vi "image acquisition practice2fail.vi"() -> ()   [LabVIEW 2014]
uses:
  <vilib>/vision/Image Controls.llb/IMAQ Image.ctl
panel:
  out "Circular Particles":T1
  out "Image Acquired":T1(plugin-control)
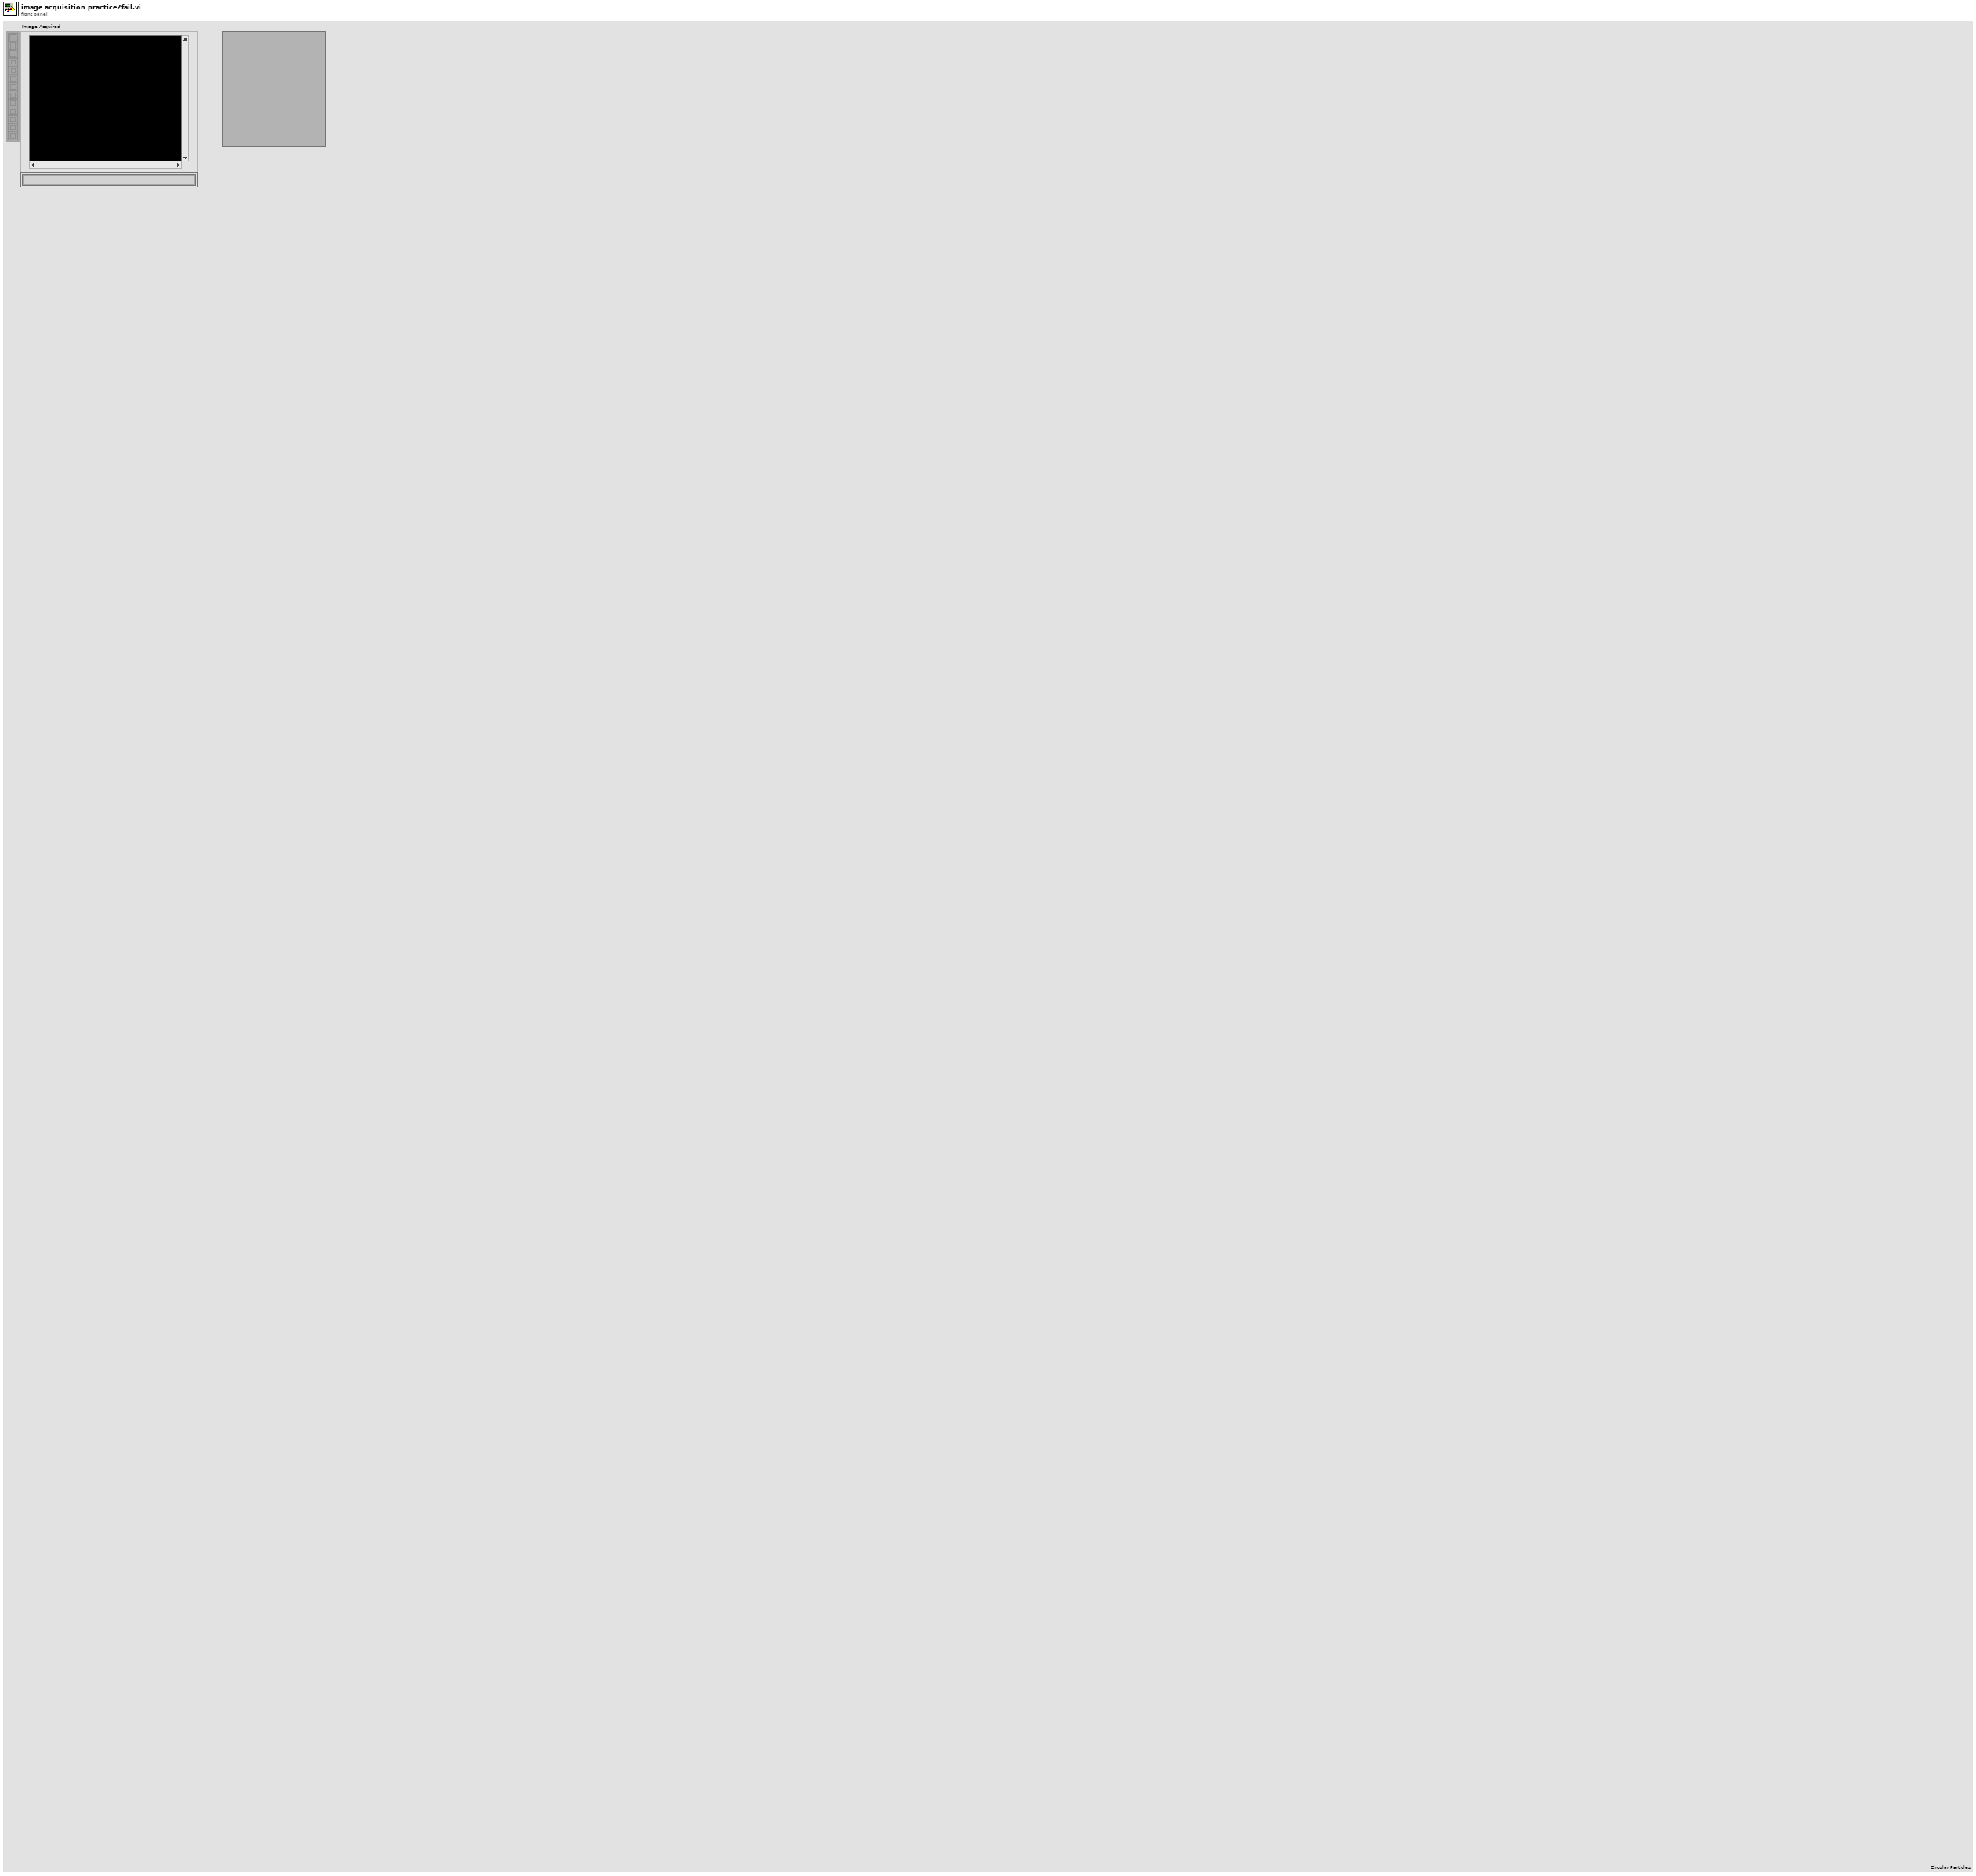
[diagram p1: front panel]
types:
  T1 = typedef "IMAQ Image.ctl" = refnum<image>
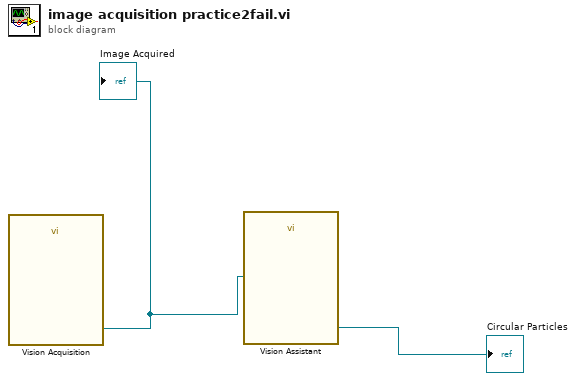
[diagram p0: block diagram]
diagram:
  n1 = call "Vision Acquisition"() -> ("Image Out"=w2:T1)  [unwired: 26 in, 1 out]
  "Image Acquired" <- w2
  n2 = call "Vision Assistant"("Image In"=w2) -> ("Image Out"=→"Circular Particles":T1)  [unwired: 25 in, 1 out]
